vi "2D limits response.vi"(7 "starting 2D state":T3, 11 "coefficient of restitution [0.9]":dbl=0.9 min=0.0 max=1.0 step=0.001, 13 "2D limits":T1) -> (8 "ending 2D state":T3)   [LabVIEW 2016]
doc: "This subVI handles the reflection off of the lower and upper limits of a box in 2D.\n\nPaul K Dixon\nP350\nCSUSB"
uses:
  typedef/2d state.ctl
  typedef/1d state.ctl
  typedef/2d limits.ctl
  typedef/1d limits.ctl
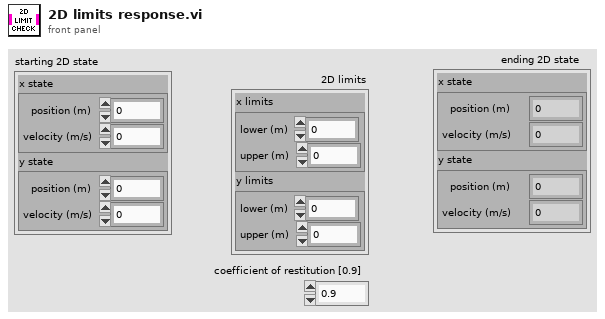
[diagram p1: front panel]
types:
  T1 = typedef "2d limits.ctl" = cluster{"x limits":T2, "y limits":T2}
  T2 = typedef "1d limits.ctl" = cluster{"lower (m)":dbl, "upper (m)":dbl}
  T3 = typedef "2d state.ctl" = cluster{"x state":T4, "y state":T4}
  T4 = typedef "1d state.ctl" = cluster{"position (m)":dbl, "velocity (m/s)":dbl}
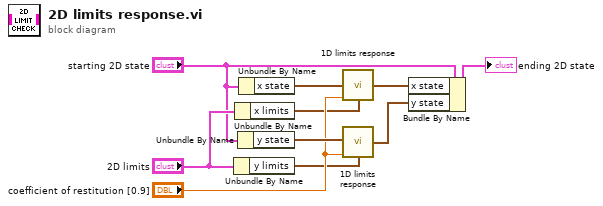
[diagram p0: block diagram]
diagram:
  n1 = Unbundle By Name("2D limits") -> ("y limits"=w6:T2)
  n2 = Unbundle By Name("2D limits") -> ("x limits"=w7:T2)
  n3 = Unbundle By Name("starting 2D state") -> ("y state"=w9:T4)
  n4 = Unbundle By Name("starting 2D state") -> ("x state"=w10:T4)
  n5 = call "1D limits response.vi"("starting state"=w10, "coefficient of restitution [0.9]"="coefficient of restitution [0.9]", "1D limits"=w7) -> ("ending state"=w2:T4)  [unwired: 12 in]
  n6 = call "1D limits response.vi"("starting state"=w9, "coefficient of restitution [0.9]"="coefficient of restitution [0.9]", "1D limits"=w6) -> ("ending state"=w1:T4)  [unwired: 12 in]
  n7 = Bundle By Name(cluster="starting 2D state", "x state"=w2, "y state"=w1) -> (→"ending 2D state":T3)
